vi "load.vi"(8 "error in (no error)":errorcluster, 10 "functional":refnum<user-event>, 11 "interface in":refnum<class "interface.lvclass">=refnum) -> (0 "error out":errorcluster, 3 "interface out":refnum<class "interface.lvclass">)   [LabVIEW 2015, in "example_01.lvlib" / "functional.lvlib" / "interface.lvclass"]
uses:
  interface.lvclass
  _controls/event_functional.ctl
  _controls/event_functional_command.ctl
  functional.lvlib
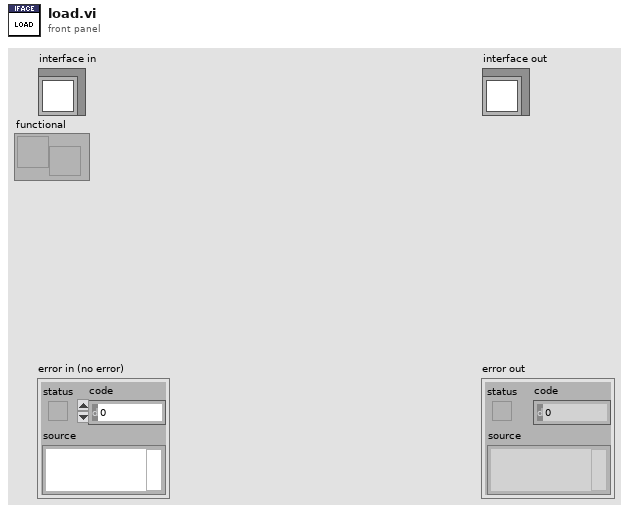
[diagram p1: front panel]
types:
  T1 = typedef "example_01.lvlib/functional.lvlib/event_functional.ctl" = cluster{"command":T2, "data":variant}
  T2 = typedef "example_01.lvlib/functional.lvlib/event_functional_command.ctl" = enum16{"<command_functional>", "--high-level", "stop", "update_hmi_references", "load_interface", "--functional", "do_it", "<null>"}
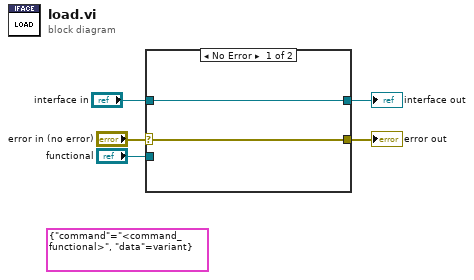
[diagram p0: block diagram]
diagram:
  (unwired) T1 {"command"=enum."<command_functional>", "data"=variant} ("event data")
  n1 = case shown="No Error" "error in (no error)" {
    selector: "error in (no error)" -> [w6 w9]
    tunnel: [w6 w9] -> w4
    tunnel: [w7 w8] -> w2
    tunnel: "interface in" -> [w7 w8]
    tunnel: "functional" -> [_ _]
    frame No Error {
    }
    frame Error {
    }
  }
  "error out" <- w4
  "interface out" <- w2
